vi "LoadDebugServerConfig.vi"(8 "error in (no error)":errorcluster) -> (0 "error out":errorcluster, 1 "Config":T1, 2 "Port":u16, 3 "Debug config path":path, 5 "Allow Remote?":bool)   [LabVIEW 2016]
uses:
  <vilib>/WebServerConfig/Config.ctl
  <vilib>/WebServerConfig/Server.ctl
  <vilib>/WebServerConfig/Alias.ctl
  <vilib>/WebServerConfig/ErrorDocument.ctl
  <vilib>/WebServerConfig/Action.ctl
  <vilib>/WebServerConfig/Redirect.ctl
  <vilib>/WebServerConfig/Interface.ctl
  <vilib>/WebServerConfig/AddHandler.ctl
  <vilib>/WebServerConfig/SSL.ctl
  <vilib>/WebServerConfig/CustomLog.ctl
  <vilib>/WebServerConfig/LoadModule.ctl
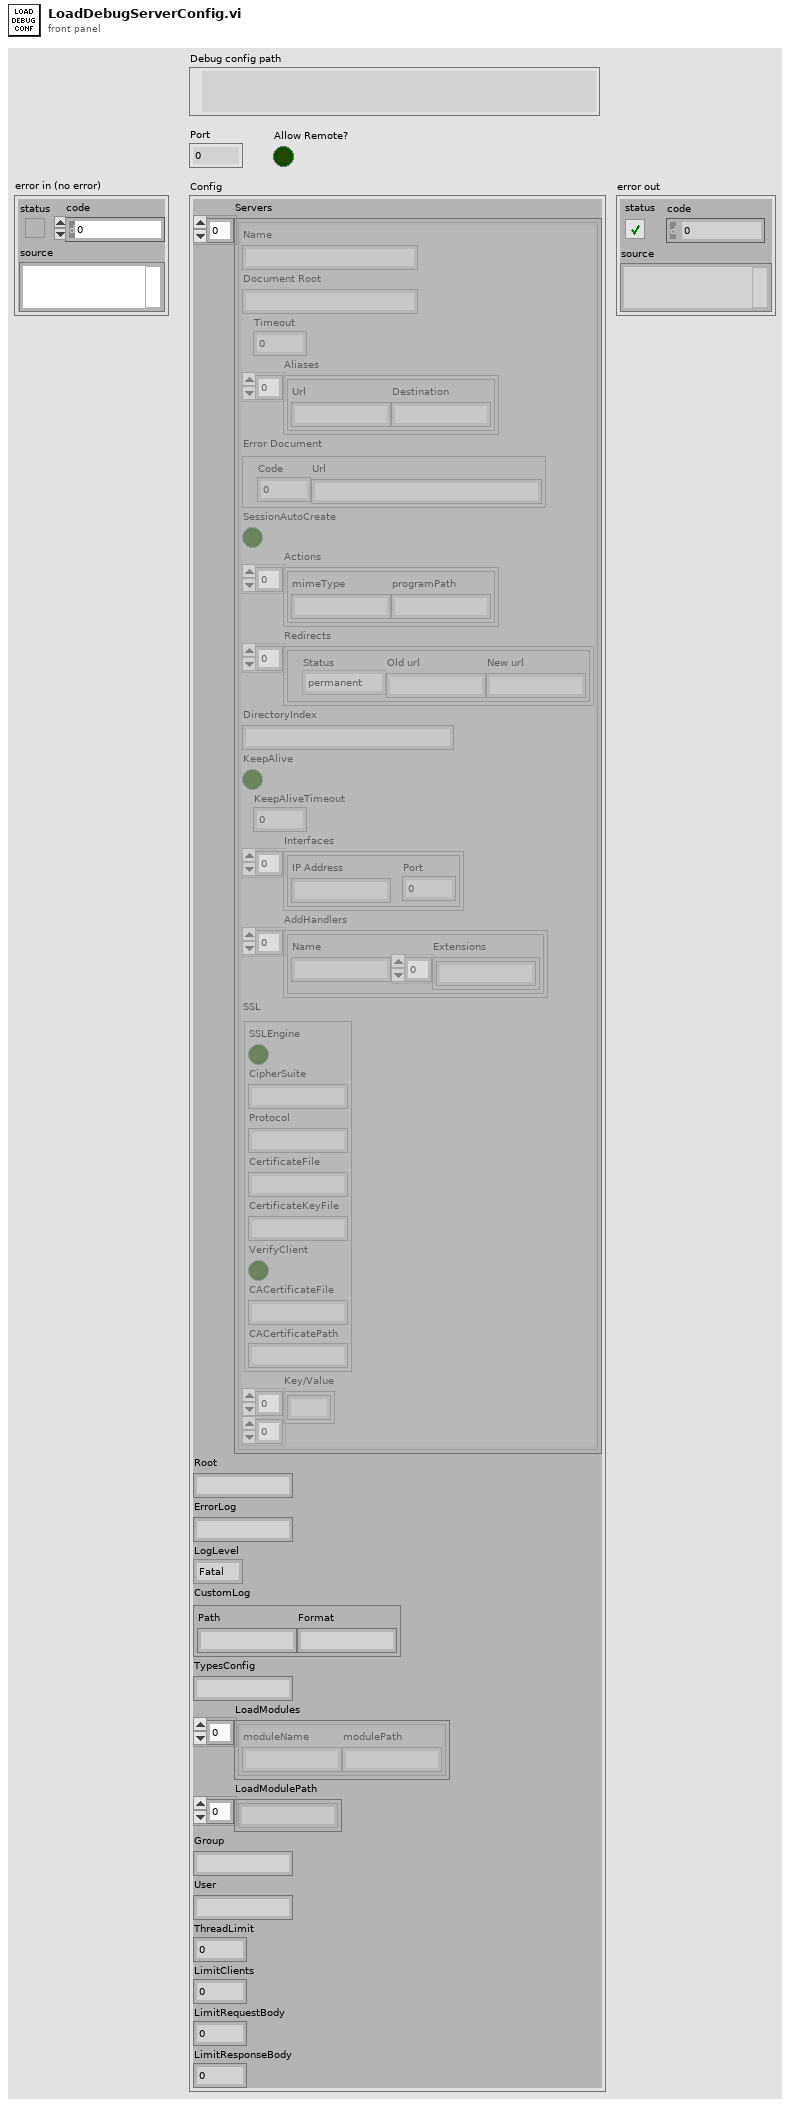
[diagram p1: front panel]
types:
  T1 = typedef "Config.ctl" = cluster{"Servers":T2[], "Root":string, "ErrorLog":string, "LogLevel":enum16{"Fatal", "Error", "Warn", "Info", "Debug", "5", "6", "7", "8", "Verbose"}, "CustomLog":T10, "TypesConfig":string, "LoadModules":T11[], "LoadModulePath":string[], "Group":string, "User":string, "ThreadLimit":u32, "LimitClients":u32, "LimitRequestBody":u32, "LimitResponseBody":u32}
  T2 = typedef "Server.ctl" = cluster{"Name":string, "Document Root":string, "Timeout":u32, "Aliases":T3[], "Error Document":T4, "SessionAutoCreate":bool, "Actions":T5[], "Redirects":T6[], "DirectoryIndex":string, "KeepAlive":bool, "KeepAliveTimeout":u32, "Interfaces":T7[], "AddHandlers":T8[], "SSL":T9, "Key/Value":string[][]}
  T3 = typedef "Alias.ctl" = cluster{"Url":string, "Destination":string}
  T4 = typedef "ErrorDocument.ctl" = cluster{"Code":u16, "Url":string}
  T5 = typedef "Action.ctl" = cluster{"mimeType":string, "programPath":string}
  T6 = typedef "Redirect.ctl" = cluster{"Status":enum16{"permanent", "temp", "seeother", "gone"}, "Old url":string, "New url":string}
  T7 = typedef "Interface.ctl" = cluster{"IP Address":string, "Port":u16}
  T8 = typedef "AddHandler.ctl" = cluster{"Name":string, "Extensions":string[]}
  T9 = typedef "SSL.ctl" = cluster{"SSLEngine":bool, "CipherSuite":string, "Protocol":string, "CertificateFile":string, "CertificateKeyFile":string, "VerifyClient":bool, "CACertificateFile":string, "CACertificatePath":string}
  T10 = typedef "CustomLog.ctl" = cluster{"Path":string, "Format":string}
  T11 = typedef "LoadModule.ctl" = cluster{"moduleName":string, "modulePath":string}
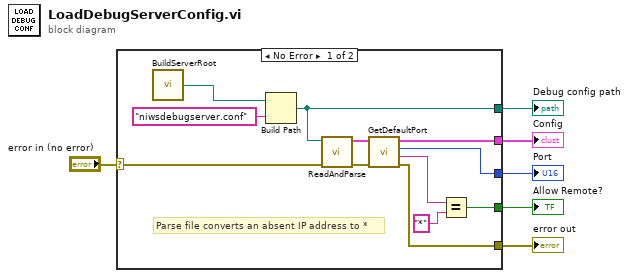
[diagram p0: block diagram]
diagram:
  n1 = case shown="No Error" "error in (no error)" {
    selector: "error in (no error)" -> [w11 w19]
    tunnel: [w18 _] -> w6
    tunnel: [w17 _] -> w5
    tunnel: [w16 _] -> w4
    tunnel: [w10 w19] -> w2
    tunnel: [w8 _] -> w1
    frame No Error {
      # "Parse file converts an absent IP address to *"
      n2 = call <vilib>:"BuildServerRoot.vi"() -> ("Server Root"=w12:path)
      n3 = Build Path(base path=w12, name or relative path="niwsdebugserver.conf") -> (appended path=w18:path)
      n4 = call <vilib>:"ReadAndParse.vi"("error in (no error)"=w11, "Path"=w18) -> ("error out"=w15:errorcluster, "Config"=w14:T1)  [unwired: 8 in]
      n5 = call <resource>:"GetDefaultPort.vi"("error in (no error)"=w15, "Config in"=w14) -> ("error out"=w10:errorcluster, "IP Address"=w9:string, "Port"=w16:u16, "Config out"=w17:T1)  [unwired: 6 in]
      n6 = Equal?(x=w9, y="*" ("x")) -> (x = y?=w8:bool)
    }
    frame Error {
    }
  }
  "Debug config path" <- w6
  "Config" <- w5
  "Port" <- w4
  "error out" <- w2
  "Allow Remote?" <- w1
